vi "5p1_HW_Task1B_jones6sv.vi"() -> ()   [LabVIEW 2016]
uses:
  <vilib>/express/express arith-compare/Formula/XNode/ExpressFormulaBlockNode.xnode
panel:
  out "Stopping sight distance":dbl caption="Stopping sight distance (S)(ft)"
  in  "Reaction time (TR)":dbl
  in  "Up or down hill (+ or -)":string(combo)
  in  "Grade of road (G)":dbl
  in  "Friction (F)":dbl
  in  "Vehicle speed (V)":dbl
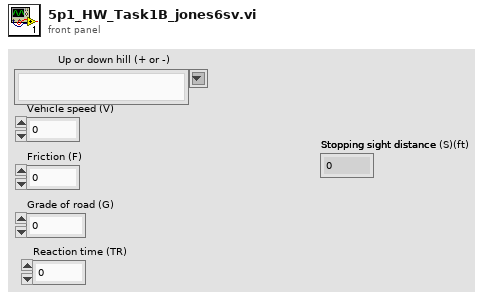
[diagram p1: front panel]
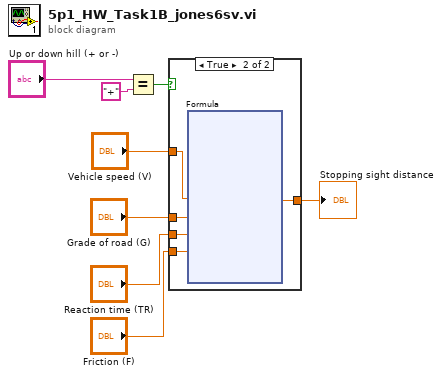
[diagram p0: block diagram]
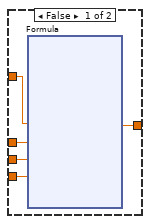
[diagram p2: hidden frame]
diagram:
  n1 = Equal?(x="Up or down hill (+ or -)", y="+" ("String")) -> (x = y?=w6:bool)
  n2 = case shown="True" w6 {
    tunnel: "Grade of road (G)" -> [w13 w31]
    tunnel: "Reaction time (TR)" -> [w12 w32]
    tunnel: "Vehicle speed (V)" -> [w11 w30]
    tunnel: [w10 w29] -> w2
    tunnel: "Friction (F)" -> [w9 w28]
    frame False {
      n3 = xnode "Formula"("V"=w11, "G"=w13, "TR"=w12, "F"=w9) -> ("Result"=w10:dbl)  [unwired: 1 in, 1 out]
    }
    frame True {
      n4 = xnode "Formula"("V"=w30, "G"=w31, "TR"=w32, "F"=w28) -> ("Result"=w29:dbl)  [unwired: 1 in, 1 out]
    }
  }
  "Stopping sight distance" <- w2
